vi "数据写入入队列 (子VI).vi"   [LabVIEW 2016, in "斯坦道CODMn.lvlib"]
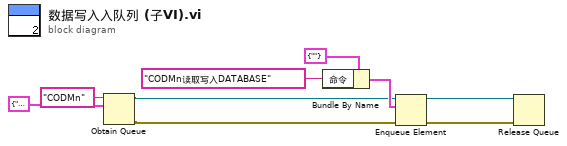
[diagram p0: block diagram]
diagram:
  n1 = Obtain Queue(name (unnamed)="CODMn" ("名称（未命名）"), element data type=cluster{"命令":string} {"命令"="启用模块"} ("元素")) -> (queue out=w4:refnum<queue>, error out=w3:errorcluster)  [unwired: 3 in, 1 out]
  n2 = Bundle By Name(cluster=cluster{"命令":string} {"命令"=""} ("元素"), "命令"="CODMn读取写入DATABASE" ("名称（未命名）")) -> (w5:cluster{"命令":string})
  n3 = Enqueue Element(queue=w4, element=w5, error in (no error)=w3) -> (queue out=w2:refnum<queue>, error out=w1:errorcluster)  [unwired: 1 in, 1 out]
  n4 = Release Queue(queue=w2, error in (no error)=w1) -> ()  [unwired: 1 in, 3 out]
